vi "Zoom_FaktorAndorNull.vi"(8 "error in (no error)":errorcluster, 9 "Limit to 1x":bool, 10 "Array":bool[](array[boolean]), 11 "ZoomInteger 2":cluster{"X":i32, "Y":i32}) -> (0 "error out":errorcluster, 2 "X":dbl, 3 "ZoomInteger":cluster{"X":i32, "Y":i32})   [LabVIEW 2011]
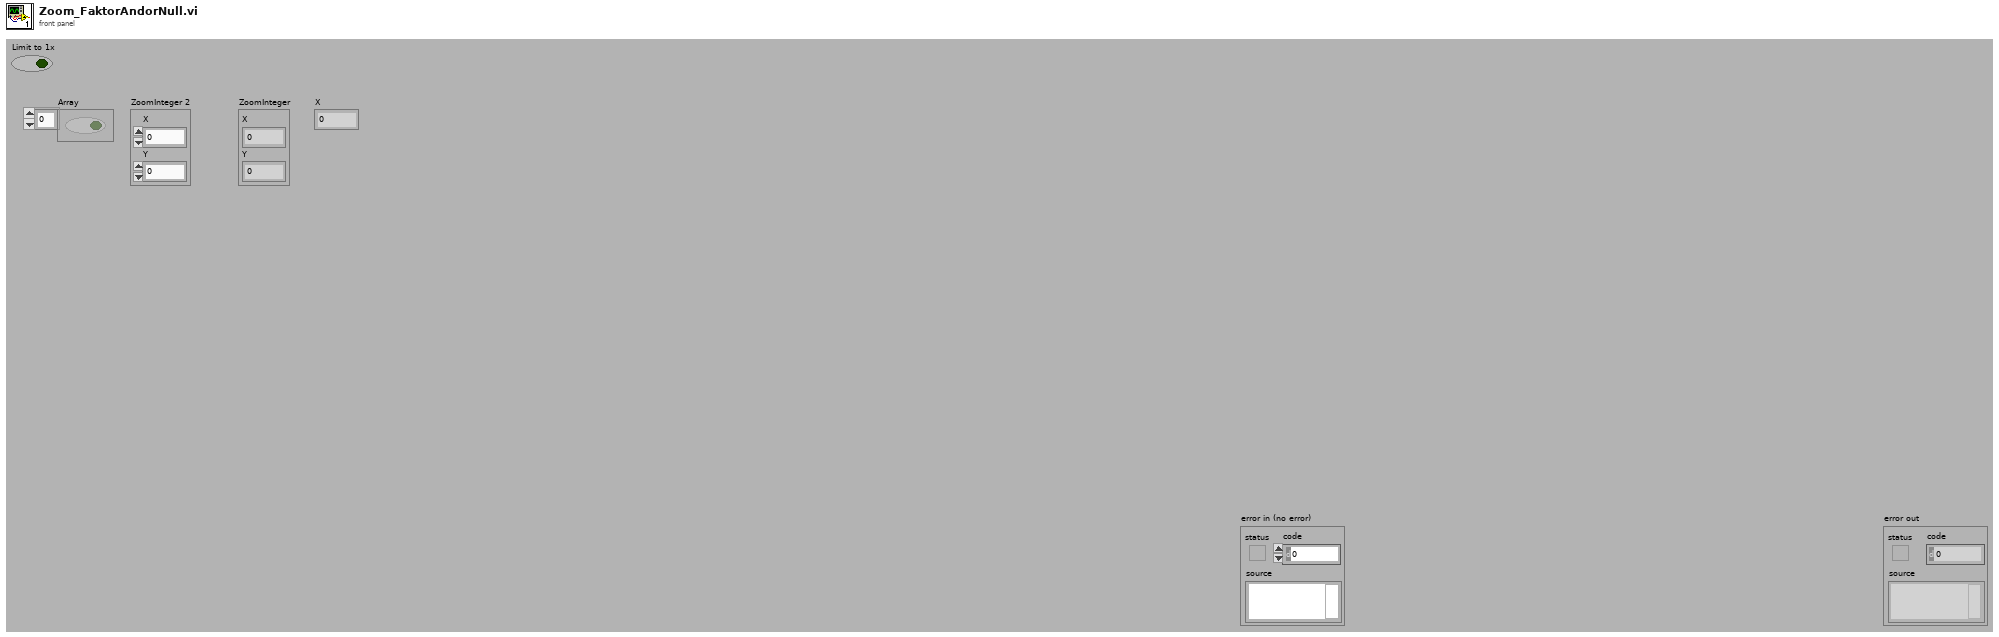
[diagram p1: front panel]
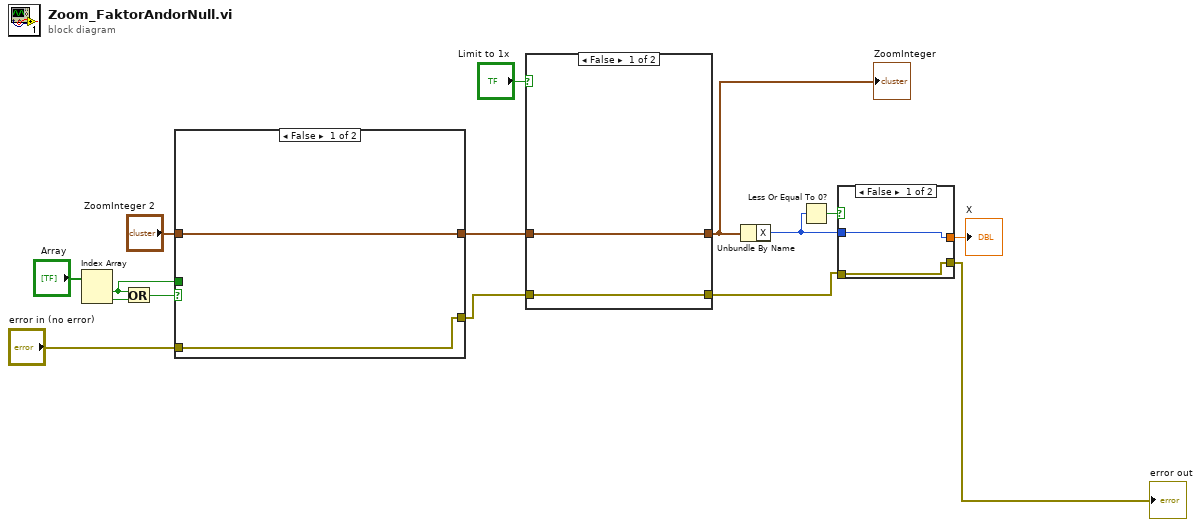
[diagram p0: block diagram]
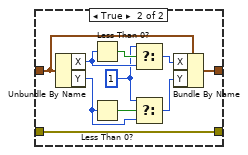
[diagram p2: hidden frame]
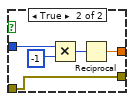
[diagram p3: hidden frame]
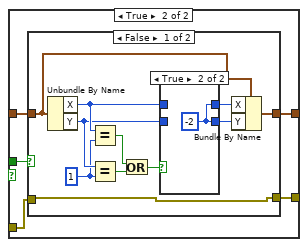
[diagram p4: hidden frame]
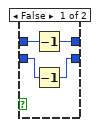
[diagram p5: hidden frame]
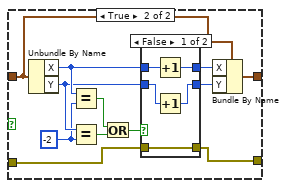
[diagram p6: hidden frame]
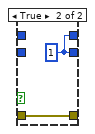
[diagram p7: hidden frame]
diagram:
  n1 = Index Array(array="Array") -> (element #1=w15:bool, element #2=w14:bool)  [unwired: 2 in]
  n2 = Or(x=w15, y=w14) -> (x .or. y?=w8:bool)
  n3 = case shown="False" w8 {
    tunnel: w15 -> [_ w22]
    tunnel: "ZoomInteger 2" -> [w17 w21]
    tunnel: [w17 w20] -> w7
    tunnel: "error in (no error)" -> [w16 w19]
    tunnel: [w16 w18] -> w3
    frame False {
    }
    frame True {
      n4 = case shown="False" w22 {
        tunnel: w21 -> [w25 w47]
        tunnel: [w24 w48] -> w20
        tunnel: w19 -> [w23 w40]
        tunnel: [w23 w39] -> w18
        frame False {
          w29 = 1 ("y")
          n5 = Unbundle By Name(w25) -> ("X"=w31:i32, "Y"=w30:i32)
          n6 = Equal?(x=w31, y=w29) -> (x = y?=w28:bool)
          n7 = Equal?(x=w30, y=w29) -> (x = y?=w27:bool)
          n8 = Or(x=w28, y=w27) -> (x .or. y?=w26:bool)
          n9 = case shown="True" w26 {
            tunnel: [w37 w38] -> w33
            tunnel: [w36 w38] -> w32
            tunnel: w31 -> [w35 _]
            tunnel: w30 -> [w34 _]
            frame False {
              n10 = Decrement(x=w35) -> (x-1=w37:i32)
              n11 = Decrement(x=w34) -> (x-1=w36:i32)
            }
            frame True {
              w38 = -2
            }
          }
          n12 = Bundle By Name(cluster=w25, "X"=w33, "Y"=w32) -> (w24:cluster{"X":i32, "Y":i32})
        }
        frame True {
          w44 = -2 ("y")
          n13 = Unbundle By Name(w47) -> ("X"=w46:i32, "Y"=w45:i32)
          n14 = Equal?(x=w46, y=w44) -> (x = y?=w43:bool)
          n15 = Equal?(x=w45, y=w44) -> (x = y?=w42:bool)
          n16 = Or(x=w43, y=w42) -> (x .or. y?=w41:bool)
          n17 = case shown="False" w41 {
            tunnel: [w55 w57] -> w50
            tunnel: [w54 w57] -> w49
            tunnel: w46 -> [w53 _]
            tunnel: w45 -> [w52 _]
            tunnel: w40 -> [w51 w56]
            tunnel: [w51 w56] -> w39
            frame False {
              n18 = Increment(x=w53) -> (x+1=w55:i32)
              n19 = Increment(x=w52) -> (x+1=w54:i32)
            }
            frame True {
              w57 = 1
            }
          }
          n20 = Bundle By Name(cluster=w47, "X"=w50, "Y"=w49) -> (w48:cluster{"X":i32, "Y":i32})
        }
      }
    }
  }
  n21 = case shown="False" "Limit to 1x" {
    tunnel: w7 -> [w59 w63]
    tunnel: [w59 w62] -> w5
    tunnel: w3 -> [w58 w60]
    tunnel: [w58 w60] -> w2
    frame False {
    }
    frame True {
      w61 = 1 ("t")
      n22 = Unbundle By Name(w63) -> ("X"=w68:i32, "Y"=w66:i32)
      n23 = Less Than 0?(x=w68) -> (x < 0?=w69:bool)
      n24 = Less Than 0?(x=w66) -> (x < 0?=w67:bool)
      n25 = Select(t=w61, s=w69, f=w68) -> (s? t:f=w65:i32)
      n26 = Select(t=w61, s=w67, f=w66) -> (s? t:f=w64:i32)
      n27 = Bundle By Name(cluster=w63, "X"=w65, "Y"=w64) -> (w62:cluster{"X":i32, "Y":i32})
    }
  }
  "ZoomInteger" <- w5
  n28 = Unbundle By Name(w5) -> ("X"=w11:i32)
  n29 = Less Or Equal To 0?(x=w11) -> (x <= 0?=w12:bool)
  n30 = case shown="False" w12 {
    tunnel: w11 -> [w71 w76]
    tunnel: [w71 w73] -> w10
    tunnel: w2 -> [w70 w72]
    tunnel: [w70 w72] -> w1
    frame False {
    }
    frame True {
      n31 = Multiply(x=w76, y=-1) -> (x*y=w74:i32)
      n32 = Reciprocal(x=w74) -> (1/x=w73:dbl)
    }
  }
  "X" <- w10
  "error out" <- w1
